vi "Global check.vi"() -> ()   [LabVIEW 2012, in "StageSPIM.lvclass"]
uses:
  StageSPIM/StageSPIM.lvclass
panel:
  in  "check if at destination?":bool
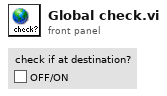
[diagram p1: front panel]
diagram:
